vi "Loop Get Input Output Assignements VHDL.vi"(10 "Inside Terms[] offset":i32, 11 "Loop Tunnels[]":refnum<vi>[](array[refnum])) -> (2 "tunnels output assignements":string, 3 "tunnesl input assignements":string)   [LabVIEW 2018]
doc: "Return C code assignement for getting input values from outside into Loop and also assign values to outside wires.\nInside Terms[] offset is for multiframe structures (CaseStructure),it's used when parsing tunnels to use right internal terminal, because each outside terminal has N inside terminals (N is count of structure frames)."
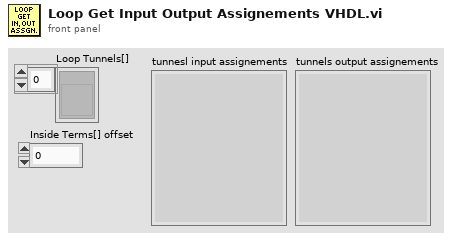
[diagram p1: front panel]
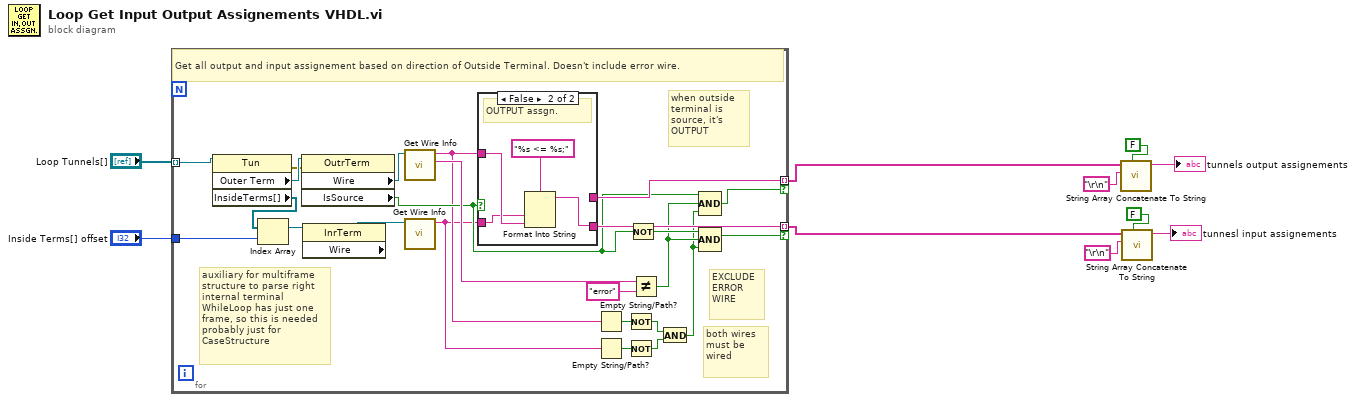
[diagram p0: block diagram]
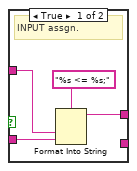
[diagram p2: hidden frame]
diagram:
  n1 = for {
    tunnel: "Loop Tunnels[]" -> [w32] mode=indexing
    tunnel: [w28] -> w2 mode=indexing if=w26
    tunnel: [w27] -> w1 mode=indexing if=w25
    tunnel: "Inside Terms[] offset" -> [w21]
    # "auxiliary for multiframe structure to parse right internal terminal\nWhileLoop has just one frame, so this is needed probably just for CaseStructure"
    # "both wires must be wired"
    # "EXCLUDE ERROR WIRE"
    # "when outside terminal is source, it's OUTPUT"
    # "Get all output and input assignement based on direction of Outside Terminal. Doesn't include error wire."
    n2 = property class="Tun"(reference=w32) -> (error out=w33:errorcluster, "Outer Term"=w34:refnum<vi>, "InsideTerms[]"=w11:refnum<vi>[])  [unwired: 1 in, 1 out]
    n3 = Index Array(array=w11, index=w21) -> (element=w30:refnum<vi>)
    n4 = property class="OutrTerm"(reference=w34, error in=w33) -> ("Wire"=w31:refnum<vi>, "IsSource"=w19:bool)  [unwired: 2 out]
    n5 = property class="InrTerm"(reference=w30) -> ("Wire"=w29:refnum<vi>)  [unwired: 1 in, 2 out]
    n6 = call "Get Wire Info.vi"("Wire"=w31) -> ("wire datatype"=w20:string, "wire label"=w17:string)  [unwired: 9 in]
    n7 = call "Get Wire Info.vi"("Wire"=w29) -> ("wire label"=w15:string)  [unwired: 9 in, 1 out]
    n8 = case shown="False" w19 {
      tunnel: w17 -> [w37 w41]
      tunnel: w15 -> [w36 w40]
      tunnel: [w35 _] -> w28
      tunnel: [_ w39] -> w27
      frame True {
        # "INPUT assgn."
        n9 = Format Into String(format string="%s <= %s;", w37, w36) -> (resulting string=w35:string)  [unwired: 2 in, 1 out]
      }
      frame False {
        # "OUTPUT assgn."
        n10 = Format Into String(format string="%s <= %s;", w40, w41) -> (resulting string=w39:string)  [unwired: 2 in, 1 out]
      }
    }
    n11 = Empty String/Path?(string/path=w17) -> (empty?=w18:bool)
    n12 = Empty String/Path?(string/path=w15) -> (empty?=w16:bool)
    n13 = Not(x=w18) -> (.not. x?=w14:bool)
    n14 = Not(x=w16) -> (.not. x?=w13:bool)
    n15 = Not(x=w19) -> (.not. x?=w24:bool)
    n16 = Not Equal?(x=w20, y="error") -> (x != y?=w23:bool)
    n17 = And(x=w14, y=w13) -> (x .and. y?=w12:bool)
    n18 = Compound Arithmetic op=AND(w19, w23, w12) -> (w26:bool)
    n19 = Compound Arithmetic op=AND(w24, w23, w12) -> (w25:bool)
  }
  n20 = call "String Array Concatenate To String.vi"("insert last delimiter?"=FALSE, "Delimiter char"="\r\n", "Array String In"=w2) -> ("String"=→"tunnels output assignements":string)  [unwired: 8 in]
  n21 = call "String Array Concatenate To String.vi"("insert last delimiter?"=FALSE, "Delimiter char"="\r\n", "Array String In"=w1) -> ("String"=→"tunnesl input assignements":string)  [unwired: 8 in]
